vi "错误代码.vi"() -> (3 "Status_Read":u32)   [LabVIEW 2020]
uses:
  Libraries/S7/S7.lvlib
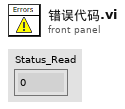
[diagram p1: front panel]
types:
  T1 = typedef "S7.lvlib/Read_Data (Reply Payload)--cluster.ctl" = cluster{"读取成功":bool, "数据":u32[], "Read_Data_error":errorcluster}
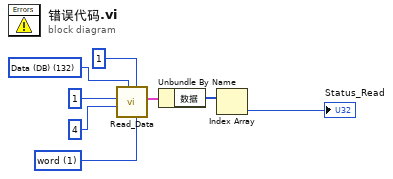
[diagram p0: block diagram]
diagram:
  w5 = u16 1 items=["byte", "word", "Dword"] ("数据类型")
  w6 = u8 132 items=["I/O (P)"=128, "Input (I)"=129, "Output (Q)"=130, "Bit Memory (M)"=131, "Data (DB)"=132, "Instance Data (DI)"=133, "Local Data (L)"=134, "Predecessor Local Data (VL)"=135] ("寄存器类型")
  n1 = call "Read_Data.vi"("数据类型"=w5, "读取长度"=u16 1, "寄存器类型"=w6, "起始地址"=u32 4, "DB #"=u16 1) -> ("Reply Payload"=w3:T1)  [unwired: 4 in, 2 out]
  n2 = Unbundle By Name(w3) -> ("数据"=w2:u32[])
  n3 = Index Array(array=w2) -> (element=→"Status_Read":u32)  [unwired: 1 in]
